vi "Pre Launch Init.vi"(11 "Assert Startup UI in":refnum<class "Assert Startup UI.lvclass">) -> (0 "error out":errorcluster, 3 "Assert Startup UI out":refnum<class "Assert Startup UI.lvclass">)   [LabVIEW 2017, in "Assert API Components.lvlib" / "Assert Startup UI.lvlib" / "Assert Startup UI.lvclass"]
doc: "(<B>Filename</B>: Actor Framework.lvlib:Actor.lvclass:Pre Launch Init.vi)\n\nDefines behavior that occurs after the Launch Nested Actor method is invoked but before the actor's Actor Core method begins running.\n\nBy default, this method does nothing. A descendant class may override it to define behavior."
uses:
  Assert Startup UI.lvclass
  <vilib>/ActorFramework/Message Enqueuer/Message Enqueuer.lvclass
  Assert Startup UI.lvclass/Assert Startup UI.ctl
  Base UI Actor/Base UI Actor/Base UI Actor.lvclass
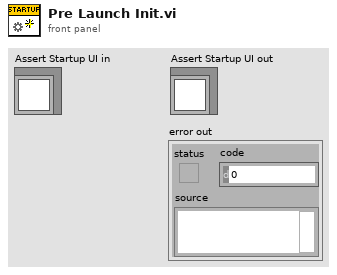
[diagram p1: front panel]
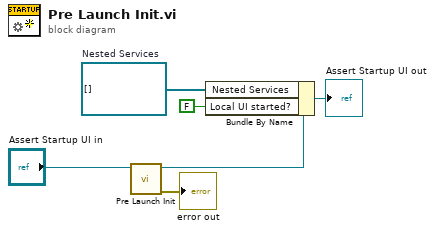
[diagram p0: block diagram]
diagram:
  w4 = refnum<class "Message Enqueuer.lvclass">[] []  # Nested Services
  n1 = call-parent "Pre Launch Init.vi"("Base UI Actor in"="Assert Startup UI in") -> ("error out"=→"error out":errorcluster, "Base UI Actor out"=w2:refnum<class "Assert Startup UI.lvclass">)  [unwired: 9 in]
  n2 = Bundle By Name(cluster=w2, "Nested Services"=w4, "Local UI started?"=FALSE) -> (→"Assert Startup UI out":refnum<class "Assert Startup UI.lvclass">)
